vi "Cliente-SAEG.vi"(11 "Boolean 2":bool) -> (1 "status":bool)   [LabVIEW 2016]
panel:
  in  "stop 2":bool
  out "Waveform Chart 2":dbl[](graph)
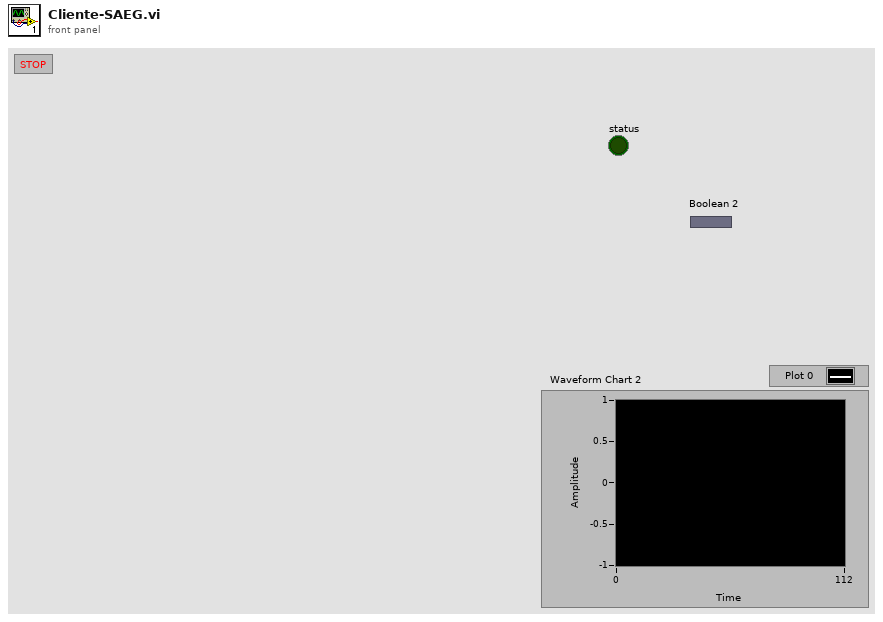
[diagram p1: front panel]
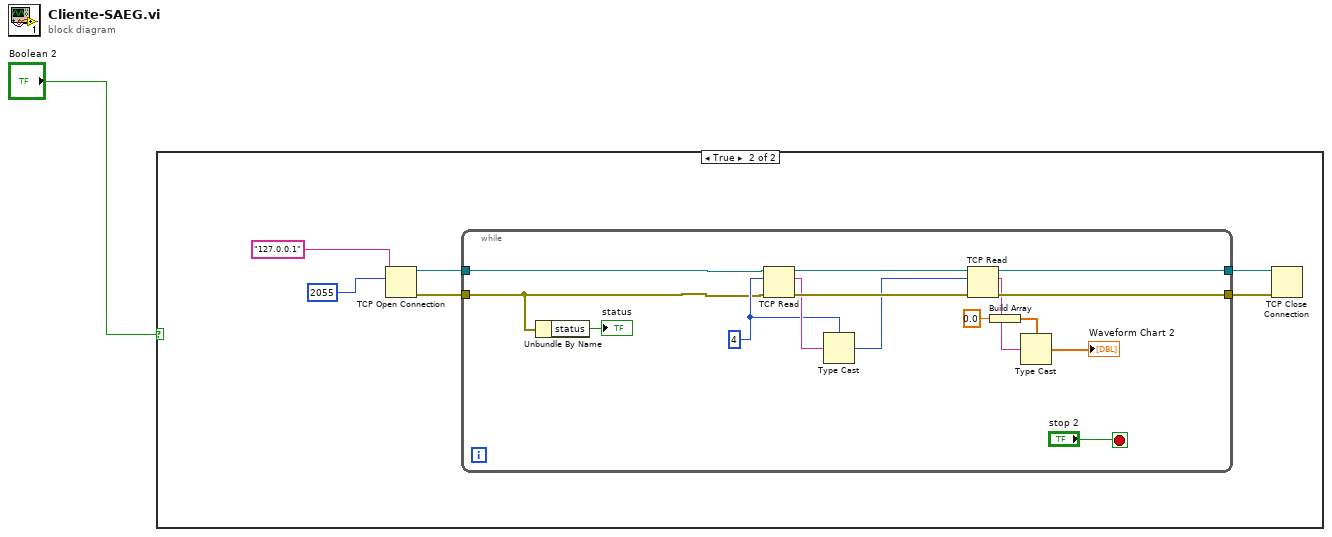
[diagram p0: block diagram]
diagram:
  n1 = case shown="True" "Boolean 2" {
    frame False {
    }
    frame True {
      n2 = TCP Open Connection(address="127.0.0.1", remote port or service name=u16 2055) -> (connection ID=w3:refnum<k5>, error out=w4:errorcluster)  [unwired: 3 in]
      n3 = while {
        tunnel: [w20] -> w2
        tunnel: w3 -> [w10]
        tunnel: w4 -> [w9]
        tunnel: [w18] -> w5
        stop <- "stop 2" stop-if-true
        w16 = 4 ("bytes to read")
        n4 = Unbundle By Name(w9) -> ("status"=→"status":bool)
        n5 = TCP Read(connection ID=w10, bytes to read=w16, error in (no error)=w9) -> (connection ID out=w22:refnum<k5>, data out=w17:string, error out=w19:errorcluster)  [unwired: 2 in]
        n6 = Type Cast(type=w16, x=w17) -> (*(type *) &x=w15:i32)
        n7 = TCP Read(connection ID=w22, bytes to read=w15, error in (no error)=w19) -> (connection ID out=w20:refnum<k5>, data out=w14:string, error out=w18:errorcluster)  [unwired: 2 in]
        n8 = Build Array(0.0 ("element")) -> (w12:dbl[])
        n9 = Type Cast(type=w12, x=w14) -> (*(type *) &x=→"Waveform Chart 2":dbl[])
      }
      n10 = TCP Close Connection(connection ID=w2, error in (no error)=w5) -> ()  [unwired: 1 in, 2 out]
    }
  }
